vi "IV2-LCRZ.vi"(0 "Voltage In":cdb=0.025284189624824437+0.006382322067092291i format="%#_4p", 1 "Test Frequency":dbl=10000.0, 2 "UseCorrection":bool, 3 "R_Shunt":dbl=25.0, 5 "Current In":cdb=1.033046760764921-0.3950958323510868i format="%#_4p", 9 "ESL":dbl=2.3e-07, 11 "ESR":dbl=0.001, 12 "Rg_VMon":dbl=5000.0 min=0.1 max=10000000000.0, 14 "Rg_IMon":dbl=5000.0 min=0.1 max=10000000000.0) -> (4 "Impedance (Mag)":dbl=0.5905262941298337 format="%#_3p", 6 "Impedance (Phase)":dbl=35.09655053885756 format="%#_3p", 8 "Inductance":dbl=5.4037341931629855e-06 format="%#_3p", 10 "Capacitance":dbl=-4.6875540145244966e-05 format="%#_3p", 15 "Real (Z)":dbl=0.483159362565652 format="%#_3p")   [LabVIEW 2020]
panel:
  out "Current Phase\nDeg":dbl=-20.929696825376666
  out "Z Phase (Pre)":dbl=35.09655053885756
  out "Z Mag (pre-correction)":dbl=0.5905262941298337
  out "VGain":dbl=5.5024763619991 format="%#_3p"
  out "Detected Current\n(Measured Signal \nmagnitude)":dbl=1.1060227514242615 format="%#_3p"
  out "I_Gain":dbl=5.512635379061372 format="%#_3p"
  out "Imag(Z)":dbl=0.3395266328638561 format="%#_3p"
  out "Voltage (mag)":dbl=0.004739188948375975 format="%#_3p"
  out "Current  (Amps)":dbl=0.008025364823694052 format="%#_3p"
  out "Voltage Phase\n (deg)":dbl=14.16685371348089 format="%.2p"
  out "Detected Voltage\n(Measured Signal\nMagnitude":dbl=0.026077275163486176 format="%.2p"
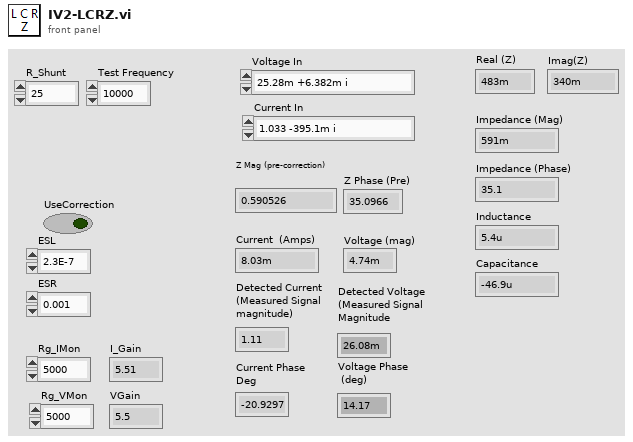
[diagram p1: front panel]
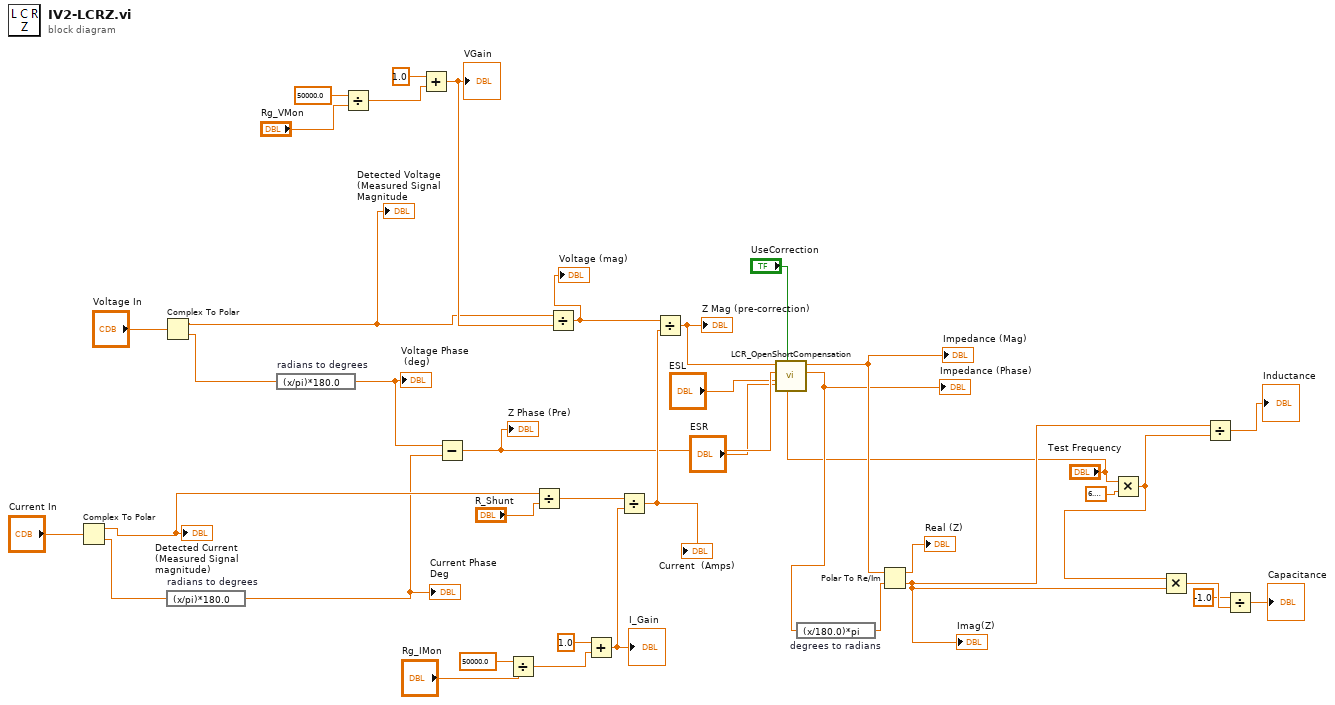
[diagram p0: block diagram]
diagram:
  n1 = Complex To Polar(r * e^(i*theta)="Current In") -> (r=w13:dbl, theta=w8:dbl)
  "Detected Current\n(Measured Signal \nmagnitude)" <- w13
  n2 = Complex To Polar(r * e^(i*theta)="Voltage In") -> (r=w14:dbl, theta=w10:dbl)
  "Detected Voltage\n(Measured Signal\nMagnitude" <- w14
  n3 = expression code="(x/pi)*180.0" "radians to degrees"(w8) -> (w7:dbl)
  "Current Phase\nDeg" <- w7
  n4 = expression code="(x/pi)*180.0" "radians to degrees"(w10) -> (w9:dbl)
  "Voltage Phase\n (deg)" <- w9
  n5 = Divide(x=50000.0, y="Rg_VMon") -> (x/y=w26:dbl)
  n6 = Add(x=1.0, y=w26) -> (x+y=w22:dbl)
  "VGain" <- w22
  n7 = Subtract(x=w9, y=w7) -> (x-y=w20:dbl)
  "Z Phase (Pre)" <- w20
  n8 = Divide(x=50000.0, y="Rg_IMon") -> (x/y=w30:dbl)
  n9 = Divide(x=w13, y="R_Shunt") -> (x/y=w29:dbl)
  n10 = Divide(x=w14, y=w22) -> (x/y=w21:dbl)
  "Voltage (mag)" <- w21
  n11 = Add(x=1.0, y=w30) -> (x+y=w28:dbl)
  "I_Gain" <- w28
  n12 = Divide(x=w29, y=w28) -> (x/y=w27:dbl)
  "Current  (Amps)" <- w27
  n13 = Divide(x=w21, y=w27) -> (x/y=w19:dbl)
  "Z Mag (pre-correction)" <- w19
  n14 = call "LCR_OpenShortCompensation.vi"("ESR"="ESR", "Freq"="Test Frequency", "UseCorrection"="UseCorrection", "ESL"="ESL", "Phase Z Meas Deg"=w20, "Mag Z Meas"=w19) -> ("Phase Z DUT"=w6:dbl, "Mag Z DUT"=w17:dbl)  [unwired: 3 in, 1 out]
  "Impedance (Mag)" <- w17
  "Impedance (Phase)" <- w6
  n15 = expression code="(x/180.0)*pi" "degrees to radians"(w6) -> (w5:dbl)
  n16 = Polar To Re/Im(2:w5, 3:w17) -> (0:w15:dbl, 1:→"Real (Z)":dbl)
  "Imag(Z)" <- w15
  n17 = Multiply(x="Test Frequency", y=6.283185307179586) -> (x*y=w37:dbl)
  n18 = Multiply(x=w37, y=w15) -> (x*y=w36:dbl)
  n19 = Divide(x=w15, y=w37) -> (x/y=→"Inductance":dbl)
  n20 = Divide(x=-1.0, y=w36) -> (x/y=→"Capacitance":dbl)
